vi "Set Initialization Data - Cam UI.vi"(8 "error in":errorcluster, 11 "Camera detection in":refnum<class "Camera detection.lvclass">) -> (0 "error out":errorcluster, 3 "Camera detection out":refnum<class "Camera detection.lvclass">)   [LabVIEW 2026, in "Camera detection.lvclass"]
doc: "In this VI you can set the initialization data of a statically-linked subWorker."
uses:
  Camera detection.lvclass
  Camera detection.lvclass/Camera detection.ctl
  C:/Program Files/National Instruments/LabVIEW 2026/vi.lib/addons/_Workers/Library/Classes/Worker/Worker.lvclass
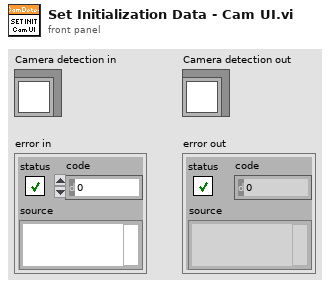
[diagram p1: front panel]
types:
  T1 = typedef "Caméra UI.lvclass/Initialization Data.ctl" = cluster{"Response Cases":T2}
  T2 = typedef "Caméra UI.lvclass/Response Cases.ctl" = cluster{"Placeholder - Can be deleted":string}
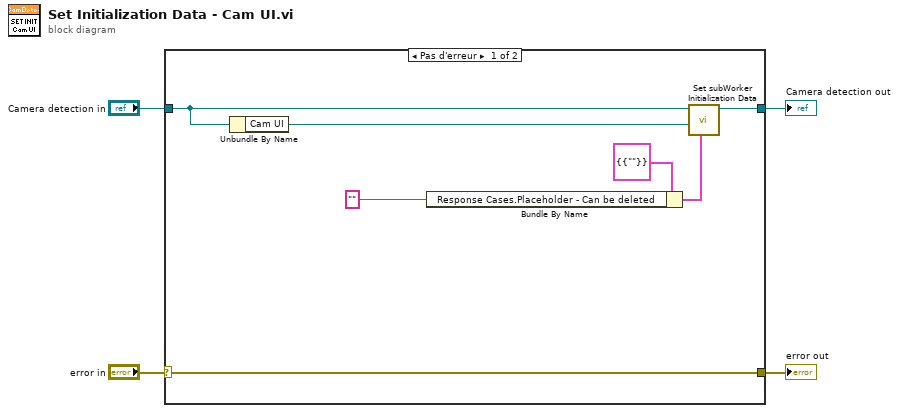
[diagram p0: block diagram]
diagram:
  n1 = case shown="Pas d'erreur" "error in" {
    selector: "error in" -> [w11 w13]
    tunnel: [w11 w13] -> w3
    tunnel: [w9 w12] -> w2
    tunnel: "Camera detection in" -> [w8 w12]
    frame No Error {
      n2 = Unbundle By Name(w8) -> ("Cam UI"=w10:refnum<class "Caméra UI.lvclass">)
      n3 = Bundle By Name(cluster=T1 {"Response Cases"={"Placeholder - Can be deleted"=""}} ("Initialization Data"), "Response Cases.Placeholder - Can be deleted"="" ("Placeholder")) -> (w6:T1)
      n4 = call-dynamic "Set subWorker Initialization Data.vi"("Initialization Data"=w6, "subWorker"=w10, "Worker"=w8) -> ("Worker out"=w9:refnum<class "Camera detection.lvclass">)  [unwired: 8 in]
    }
    frame Error {
    }
  }
  "error out" <- w3
  "Camera detection out" <- w2
